vi "GOMDBTS2048 show Config.vi"(8 "error in (no error)":errorcluster, 9 "p_controlBits":i32, 10 "p_applicationHandle":i32, 11 "handle":i32) -> (0 "error out":errorcluster, 3 "function return":i32)   [LabVIEW 2015, in "GOMDBTS2048.lvlib"]
doc: "GOBTS2048DLL int __stdcall GOMDBTS2048_showConfig(int handle, int p_applicationHandle, int p_controlBits);"
uses:
  GOMDBTS2048.lvlib
  runtime/GOMDBTS2048.dll
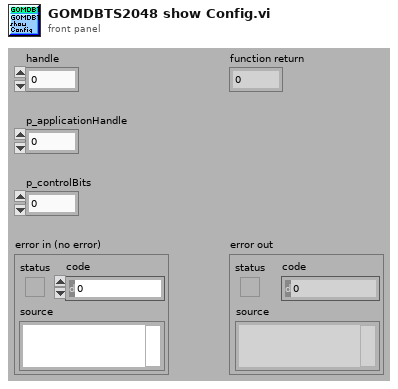
[diagram p1: front panel]
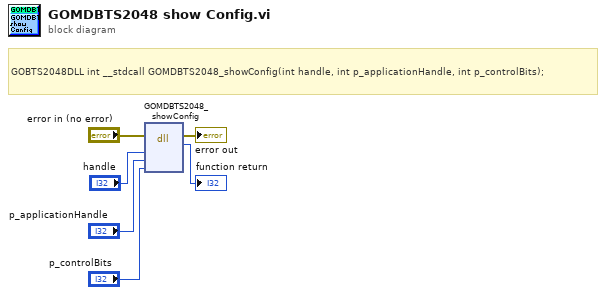
[diagram p0: block diagram]
diagram:
  # "GOBTS2048DLL int __stdcall GOMDBTS2048_showConfig(int handle, int p_applicationHandle, int p_controlBits);"
  n1 = dll-call lib="C:/Users/rkoch/Documents/GO_Library/runtime/GOMDBTS2048.*" fn="GOMDBTS2048_showConfig"(error in="error in (no error)", "handle"="handle", "p_applicationHandle"="p_applicationHandle", "p_controlBits"="p_controlBits") -> (error out=→"error out":errorcluster, →"function return":i32)  [unwired: 5 in, 1 out]
